vi "Autosend(USBCAN-2E-U).vi"(11 "CAN Device":T1={"Device Type"=20, "Device Index"=0, "CANInd"=0, "Baud(E_U)"=1835016} {"Baud(E_U)" items=["1000Kbps"=393219, "800Kbps"=393220, "500Kbps"=393223, "250Kbps"=1835016, "125Kbps"=1835025, "100Kbps"=1441827, "50Kbps"=1835052, "20Kbps"=1441971, "10Kbps"=1835232, "5Kbps"=1835457]; "Device Type" items=["PCI5121"=1, "PCI9810"=2, "USBCAN1"=3, "USBCAN2"=4, "PCI9820"=5, "PCI5110"=7, "PC104CAN"=11, "CANETUDP"=12, "PCI9840B"=14, "PC104C2"=15, "PCI9820I"=16, "CANETTCP"=17, "PCIE9221"=24, "PCI5010U"=19, "USBCAN_E_U"=20, "USBCAN_2E_U"=21, "PCI5020U"=22, "PCIE9120I"=27, "PCIE9110I"=28, "PCIE9140I"=29, "USBCAN_4E_U"=31, "USBCAN_8E_U"=34]}) -> ()   [LabVIEW 2020, in "ZLGCAN.lvclass"]
uses:
  ZLGCAN.lvclass
  Device.ctl
  ControlCAN.dll
panel:
  in  "错误输入（无错误）":errorcluster caption="Error In(No Error)"
  out "错误输出":errorcluster caption="Error Out"
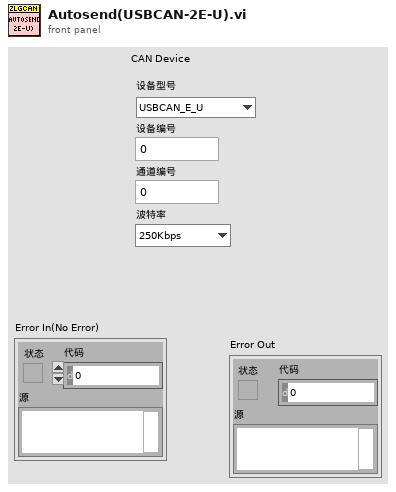
[diagram p1: front panel]
types:
  T1 = typedef "ZLGCAN.lvclass/Device.ctl" = cluster{"Device Type":u32, "Device Index":u32, "CANInd":u32, "Baud(E_U)":u32}
  T2 = cluster{u8, u8, u8, u8, u32, cluster{u32, u32, u8, u8, u8, u8, u8, u8, u8, u8, u8, u8, u8, u8, u8, u8, u8, u8}}
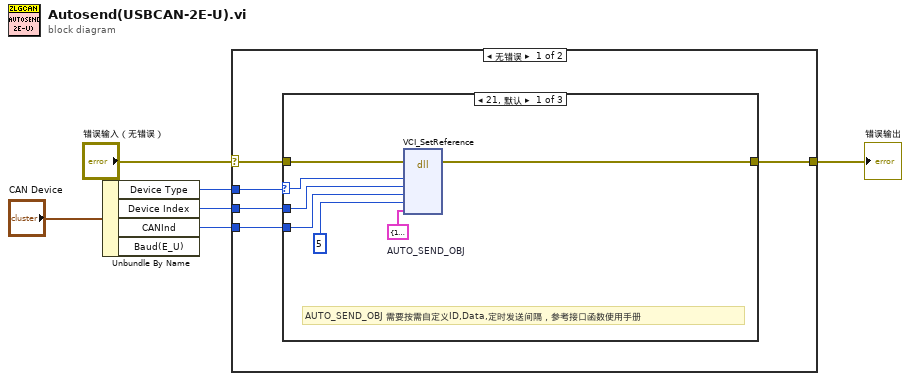
[diagram p0: block diagram]
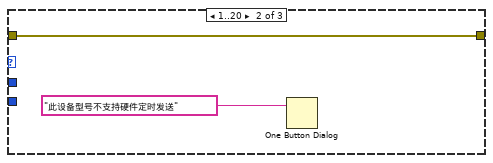
[diagram p2: hidden frame]
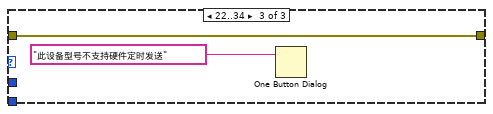
[diagram p3: hidden frame]
diagram:
  n1 = Unbundle By Name("CAN Device") -> ("Device Type"=w5:u32, "Device Index"=w4:u32, "CANInd"=w3:u32)  [unwired: 1 out]
  n2 = case shown="无错误" "错误输入（无错误）" {
    selector: "错误输入（无错误）" -> [w10 w23]
    tunnel: [w7 w23] -> w2
    tunnel: w5 -> [w11 _]
    tunnel: w4 -> [w9 _]
    tunnel: w3 -> [w8 _]
    frame No Error {
      n3 = case shown="21, 默认" w11 {
        selector: w11 -> [w16 _ _]
        tunnel: w10 -> [w18 w20 w21]
        tunnel: w9 -> [w17 _ _]
        tunnel: w8 -> [w15 _ _]
        tunnel: [w12 w20 w21] -> w7
        frame 21, Default {
          w13 = T2 {1, 0, 0, 0, 400, {17, 0, 0, 0, 0, 0, 8, 17, 17, 17, 17, 17, 17, 17, 17, 0, 0, 0}}  # AUTO_SEND_OBJ
          # "AUTO_SEND_OBJ 需要按需自定义ID,Data,定时发送间隔，参考接口函数使用手册"
          n4 = dll-call lib="PTH2sabs CUsersxu.dongDesktop新建文件夹新建文件夹 (2) - 副本ZLGCAN\nControlCANControlCAN.dll" fn="VCI_SetReference"(error in=w18, "DevType"=w16, "DevIndex"=w17, "CANInd"=w15, "RefType"=u32 5, "pData"=w13) -> (error out=w12:errorcluster)  [unwired: 7 in, 2 out]
        }
        frame 1..20 {
          n5 = One Button Dialog(message="此设备型号不支持硬件定时发送" ("消息")) -> ()  [unwired: 1 in, 1 out]
        }
        frame 22..34 {
          n6 = One Button Dialog(message="此设备型号不支持硬件定时发送" ("消息")) -> ()  [unwired: 1 in, 1 out]
        }
      }
    }
    frame Error {
    }
  }
  "错误输出" <- w2
